vi "Launch DS Server if Local URL.vi"(4 "error in (no error)":errorcluster, 6 "operation (launch)":enum16{"launch", "show", "hide", "close"}(ring), 7 "URL":string) -> (0 "error out":errorcluster, 3 "Duplicate URL":string)   [LabVIEW 2010]
doc: "If the URL input refers to the DataSocket server on this machine (for example \"dstp://localhost/wave\"), then the DataSocket server is started."
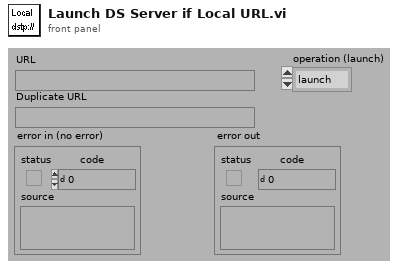
[diagram p1: front panel]
types:
  T1 = enum32{"invalid OS target", "Mac OS", "Windows 3.1", "Windows 95/NT", "Solaris 1", "Solaris 2", "HP-UX", "PowerMAX", "Linux", "Irix", "Rhapsody", "BeOS", "AIX", "OSF1", "VxWorks", "PharLap", "Carbon"}
  T2 = enum32{"invalid OS target", "Mac OS", "Windows 3.1", "Windows 95/NT", "Solaris 1", "Solaris 2", "HP-UX", "PowerMAX", "Linux", "Irix", "Rhapsody", "BeOS", "AIX", "OSF1", "VxWorks", "PharLap", "Carbon", "RTX", "Windows x64", "Linux x64"}
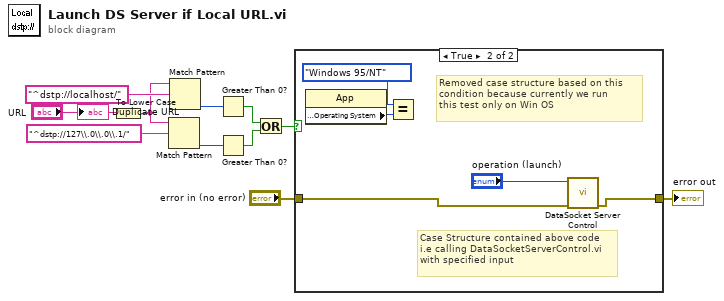
[diagram p0: block diagram]
diagram:
  n1 = To Lower Case(string="URL") -> (all lower case string=w9:string)
  n2 = Match Pattern(string=w9, regular expression="^dstp://127\\.0\\.0\\.1/") -> (offset past match=w7:i32)  [unwired: 4 out]
  n3 = Match Pattern(string=w9, regular expression="^dstp://localhost/") -> (offset past match=w8:i32)  [unwired: 4 out]
  n4 = Greater Than 0?(x=w8) -> (x > 0?=w6:bool)
  n5 = Greater Than 0?(x=w7) -> (x > 0?=w5:bool)
  n6 = Or(x=w6, y=w5) -> (x .or. y?=w4:bool)
  n7 = case shown="True" w4 {
    tunnel: "error in (no error)" -> [w12 w14]
    tunnel: [w12 w17] -> w2
    frame False {
    }
    frame True {
      # "Case Structure contained above code\ni.e calling DataSocketServerControl.vi\nwith specified input"
      # "Removed case structure based on this \ncondition because currently we run \nthis test only on Win OS"
      n8 = property class="App"() -> ("Application:Target:Operating System"=w15:T2)  [unwired: 2 in, 2 out]
      n9 = Equal?(x=T1."Windows 95/NT" ("Application:Target Operating System"), y=w15) -> ()  [unwired: 1 out]
      n10 = call <vilib>:"DataSocket Server Control.vi"("error in (no error)"=w14, "operation (launch)"="operation (launch)") -> ("error out"=w17:errorcluster)  [unwired: 5 out]
    }
  }
  "error out" <- w2
  "Duplicate URL" <- "URL"
